vi "Generate Report.vi"(6 "?":T1, 7 "report file path":path, 8 "error in (no error)":errorcluster, 9 "Write Multiple Data":T2[](array[typedef]), 10 "Image Report Setup":T3={"alignment (default)"=enum."(default)", "path or URL of image"=[], "worksheet index (0)"=1, "caption or alternative string"=[]}, 11 "template (empty)":path) -> (0 "error out":errorcluster, 2 "List Of setup":string[](array[string]))   [LabVIEW 2020]
uses:
  Control/Data Struc - Image Report Setup.ctl
  <vilib>/Utility/NIReport.llb/HTML Report Image Alignment.ctl
  Control/Data Struc -Write Multiple Data.ctl
  Control/Operation - Report Generation.ctl
  <vilib>/Utility/NIReport.llb/Report Type.ctl
  <vilib>/addons/_office/excel.llb/Excel Get Data ([str]).vi
  <vilib>/Utility/NIReport.llb/Append Image to Report (path wrap).vi
  <vilib>/Utility/NIReport.llb/Append Text Table to Report (wrap).vi
  <vilib>/Utility/NIReport.llb/NI_report.lvclass
  <vilib>/Utility/NIReport.llb/Excel/NI_Excel.lvclass
  <vilib>/addons/_office/NI_ReportGenerationToolkit.lvlib
  <vilib>/Utility/NIReport.llb/NI_ReportGenerationCore.lvlib
  Program Files (x86)/National Instruments/LabVIEW 2020/user.lib/_OpenG.lib/array/array.llb/Filter 1D Array (String)__ogtk.vi
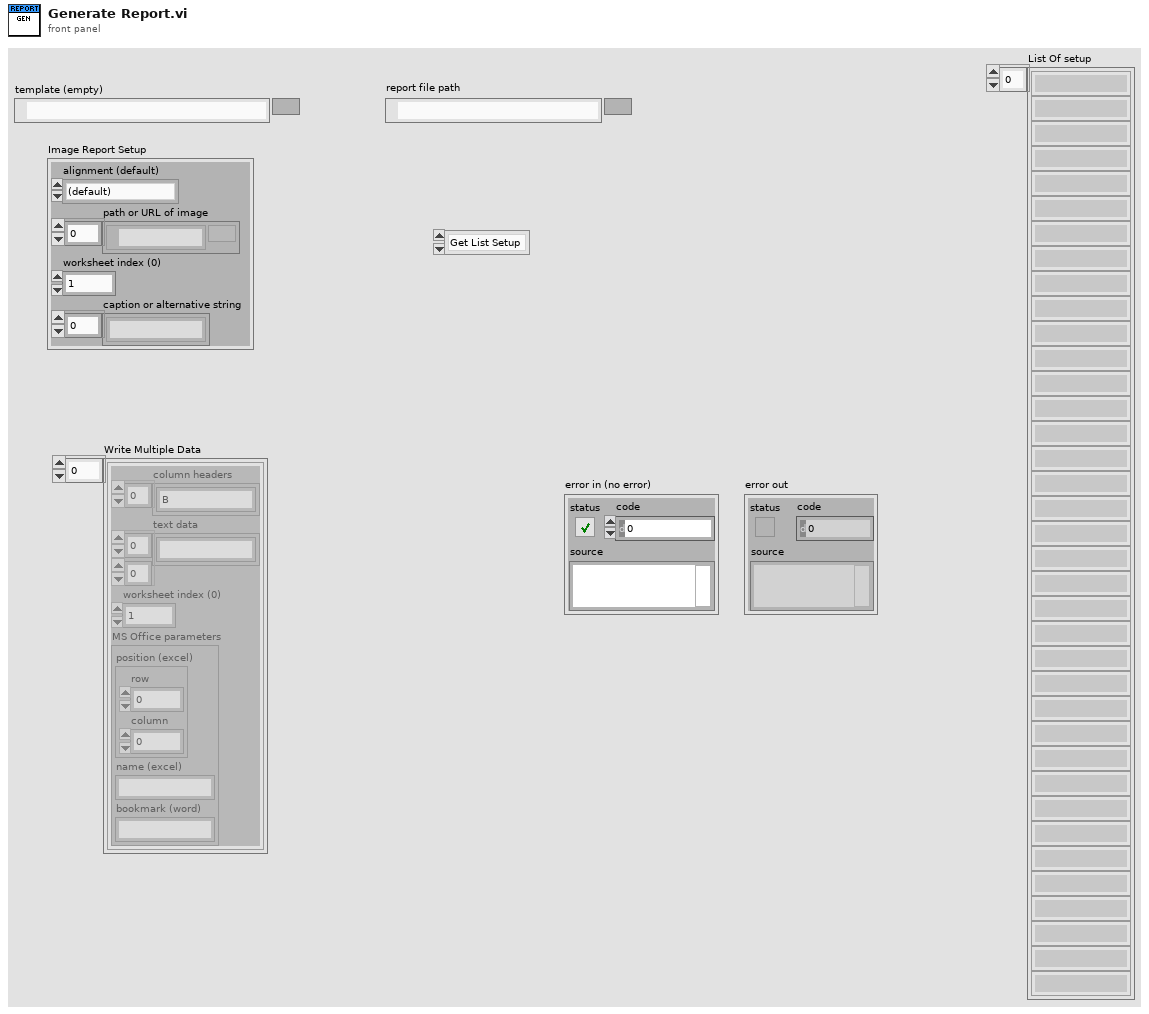
[diagram p1: front panel]
types:
  T1 = typedef "Operation - Report Generation.ctl" = enum16{"Get List Setup", "Save Image", "Generate Report"}
  T2 = typedef "Data Struc -Write Multiple Data.ctl" = cluster{"column headers":string[], "text data":string[][], "worksheet index (0)":i32, "MS Office parameters":cluster{"position (excel)":cluster{"row":i32, "column":i32}, "name (excel)":string, "bookmark (word)":string}}
  T3 = typedef "Data Struc - Image Report Setup.ctl" = cluster{"alignment (default)":T4, "path or URL of image":path[], "worksheet index (0)":i32, "caption or alternative string":string[]}
  T4 = typedef "NI_ReportGenerationCore.lvlib/HTML Report Image Alignment.ctl" = enum16{"(default)", "LEFT", "RIGHT", "TOP", "TEXTTOP", "MIDDLE", "ABSMIDDLE", "BASELINE", "BOTTOM", "ABSBOTTOM"}
  T5 = typedef "NI_ReportGenerationCore.lvlib/Report Type.ctl" = enum16{"HTML", "Word", "Excel"}
  T6 = cluster{"position (Excel)":cluster{"row":i32, "column":i32}, "name (Excel)":string, "bookmark (Word)":string}
  T7 = cluster{"position (excel)":cluster{"row":i32, "column":i32}, "name (excel)":string, "bookmark (word)":string}
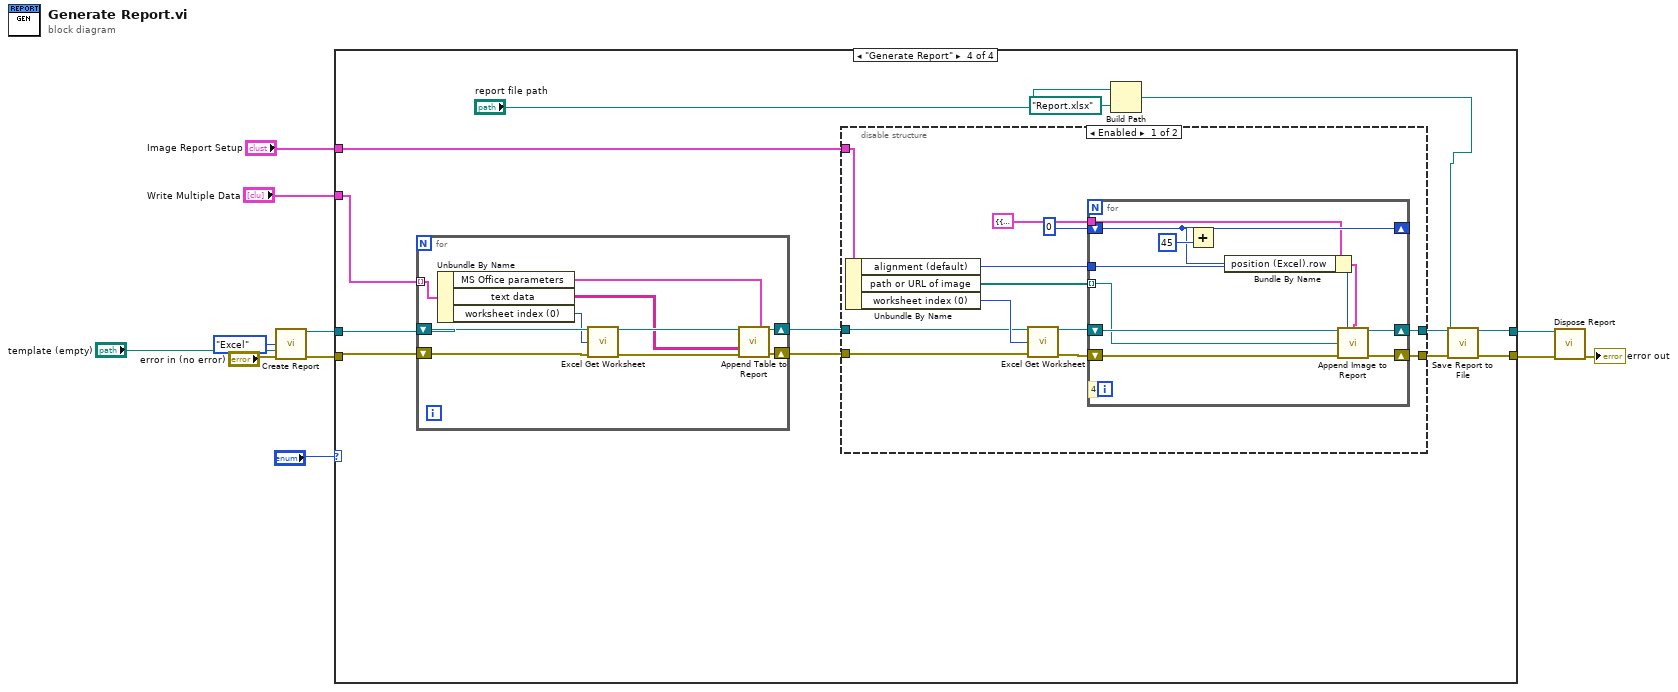
[diagram p0: block diagram]
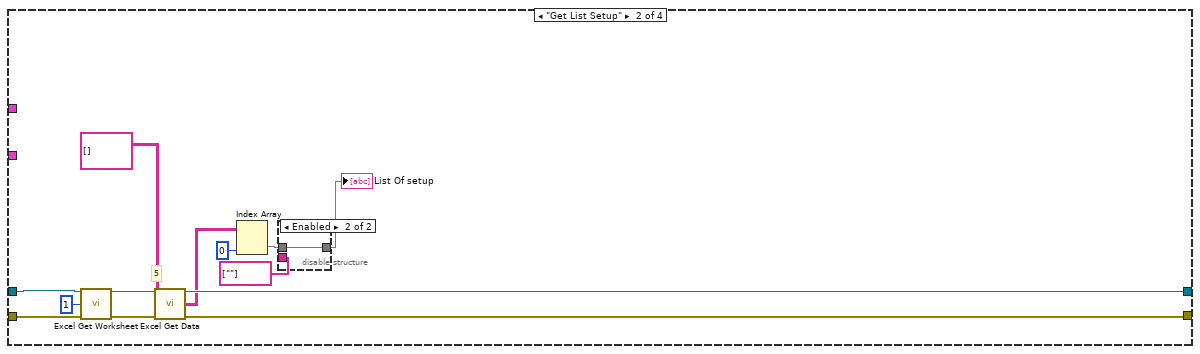
[diagram p3: hidden frame]
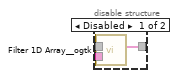
[diagram p4: hidden frame]
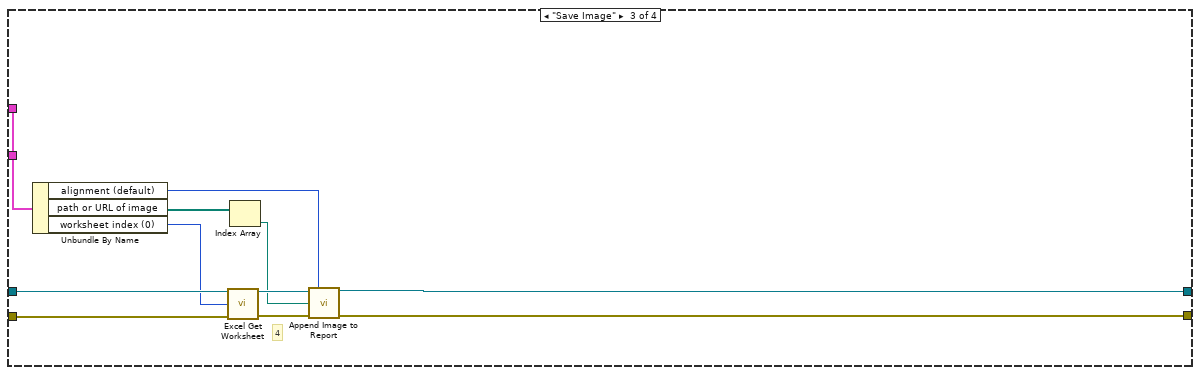
[diagram p5: hidden frame]
diagram:
  n1 = call <vilib>:"Create Report.vi"("report type"=Report_Type."Excel", "template (empty)"="template (empty)", "error in (no error)"="error in (no error)") -> ("report out"=w9:refnum<class "NI_report.lvclass">, "error out"=w11:errorcluster)  [unwired: 11 in]
  n2 = case shown="\"Generate Report\"" "?" {
    tunnel: w9 -> [w12 w21 w35 w48]
    tunnel: [w12 w20 w38 w53] -> w8
    tunnel: w11 -> [w13 w25 w40 w49]
    tunnel: [w13 w24 w41 w54] -> w10
    tunnel: "Image Report Setup" -> [_ _ w37 w50]
    tunnel: "Write Multiple Data" -> [_ _ _ w45]
    frame Default {
    }
    frame "Get List Setup" {
      # "5"
      n3 = call <vilib>:"Excel Get Worksheet.vi"("report in"=w21, "worksheet index (0)"=1, "error in (no error)"=w25) -> ("report out"=w23:refnum<class "NI_report.lvclass">, "error out"=w26:errorcluster)  [unwired: 11 out]
      n4 = call-poly <vilib>:"Excel Get Data.vi"("report in"=w23, "data type"=string[][] [], "error in (no error)"=w26) -> ("report out"=w20:refnum<class "NI_report.lvclass">, "data"=w18:string[][], "error out"=w24:errorcluster)  [unwired: 2 in, 8 out]
      n5 = Index Array(array=w18, index (col)=0 ("disabled index (col)")) -> (element=w16:string[])  [unwired: 1 in]
      n6 = disable-structure shown="Enabled" {
        disable-tunnel: w16 -> [w29 w30]
        disable-tunnel: [w28 w30] -> w15
        disable-tunnel: string[] [""] ("items to filter") -> [w27 _]
        frame Disabled {
          n7 = call-poly "Filter 1D Array__ogtk.vi"("items to filter"=w27, "array"=w29) -> ("filtered array"=w28:string[])  [unwired: 4 in, 1 out]
        }
        frame Enabled {
        }
      }
      "List Of setup" <- w15
    }
    frame "Save Image" {
      # "4"
      n8 = Unbundle By Name(w37) -> ("alignment (default)"=w36:T4, "path or URL of image"=w32:path[], "worksheet index (0)"=w33:i32)
      n9 = call <vilib>:"Excel Get Worksheet.vi"("report in"=w35, "worksheet index (0)"=w33, "error in (no error)"=w40) -> ("report out"=w34:refnum<class "NI_report.lvclass">, "error out"=w39:errorcluster)  [unwired: 11 out]
      n10 = Index Array(array=w32) -> (element=w31:path)  [unwired: 1 in]
      n11 = call-poly <vilib>:"Append Image to Report.vi"("report in"=w34, "alignment (default)"=w36, "path or URL of image"=w31, "error in (no error)"=w39) -> ("report out"=w38:refnum<class "NI_report.lvclass">, "error out"=w41:errorcluster)  [unwired: 8 in, 2 out]
    }
    frame "Generate Report" {
      n12 = for {
        shift-right: [w85] -> w47
        shift-left: w49 -> [w89]
        shift-right: [w84] -> w46
        shift-left: w48 -> [w87]
        tunnel: w45 -> [w82] mode=indexing
        n13 = Unbundle By Name(w82) -> ("MS Office parameters"=w81:T7, "text data"=w83:string[][], "worksheet index (0)"=w80:i32)
        n14 = call <vilib>:"Excel Get Worksheet.vi"("report in"=w87, "worksheet index (0)"=w80, "error in (no error)"=w89) -> ("report out"=w86:refnum<class "NI_report.lvclass">, "error out"=w88:errorcluster)  [unwired: 11 out]
        n15 = call-poly <vilib>:"Append Table to Report.vi"("report in"=w86, "MS Office parameters"=w81, "text data"=w83, "error in (no error)"=w88) -> ("report out"=w84:refnum<class "NI_report.lvclass">, "error out"=w85:errorcluster)  [unwired: 8 in, 2 out]
      }
      n16 = disable-structure shown="Enabled" {
        disable-tunnel: [w66 w79] -> w52
        disable-tunnel: [w65 w78] -> w51
        disable-tunnel: w50 -> [w64 _]
        disable-tunnel: w47 -> [w57 w78]
        disable-tunnel: w46 -> [w56 w79]
        frame Enabled {
          n17 = Unbundle By Name(w64) -> ("alignment (default)"=w63:T4, "path or URL of image"=w62:path[], "worksheet index (0)"=w61:i32)
          n18 = call <vilib>:"Excel Get Worksheet.vi"("report in"=w56, "worksheet index (0)"=w61, "error in (no error)"=w57) -> ("report out"=w55:refnum<class "NI_report.lvclass">, "error out"=w58:errorcluster)  [unwired: 11 out]
          n19 = for {
            tunnel: w63 -> [w75]
            tunnel: w62 -> [w74] mode=indexing
            shift-right: [w72] -> w65
            shift-left: w58 -> [w77]
            shift-right: [w73] -> w66
            shift-left: w55 -> [w76]
            tunnel: T6 {"position (Excel)"={"row"=0, "column"=0}, "name (Excel)"="", "bookmark (Word)"=""} ("MS Office parameters") -> [w69]
            shift-right: [w70] -> _
            shift-left: 0 -> [w68]
            # "4"
            n20 = Add(x=w68, y=45) -> (x+y=w70:i32)
            n21 = Bundle By Name(cluster=w69, "position (Excel).row"=w68) -> (w67:T6)
            n22 = call-poly <vilib>:"Append Image to Report.vi"("report in"=w76, "alignment (default)"=w75, "MS Office parameters"=w67, "path or URL of image"=w74, "error in (no error)"=w77) -> ("report out"=w73:refnum<class "NI_report.lvclass">, "error out"=w72:errorcluster)  [unwired: 7 in, 2 out]
          }
        }
        frame Disabled {
        }
      }
      n23 = Build Path(base path="report file path", name or relative path=path "Report.xlsx") -> (appended path=w42:path)
      n24 = call-dynamic "Save Report to File.vi"("report in"=w52, "report file path"=w42, "error in (no error)"=w51) -> ("report out"=w53:refnum<class "NI_report.lvclass">, "error out"=w54:errorcluster)  [unwired: 11 in]
    }
  }
  n25 = call-dynamic "Dispose Report.vi"("report in"=w8, "error in (no error)"=w10) -> ("error out"=→"error out":errorcluster)  [unwired: 13 in]
